vi "XIPIN_100G_Ethernet_1_8.vi"   [LabVIEW 2017]
doc: "The integrated 100G Ethernet IP core provides a 100G Ethernet MAC and PCS/PMA in CAUI-4, CAUI-10, or switchable CAUI-4/CAUI-10 modes, designed to the IEEE 802.3 specification. The IP supports an optional AXI4-Lite interface to access the control and status registers, high accuracy IEEE 1588v2 1-step and 2-step hardware time stamping, and a fee based IEEE 802.3bj RS-FEC core in CAUI-4 mode. For access to the integrated 100G Ethernet MAC IP, please generate a no charge license key from the 100G Ethernet product page. For access to the 100G RS-FEC core, please visit the RS-FEC product page (http://www.xilinx.com/products/intellectual-property/ef-di-100g-rs-fec.html).\n------------------------------------\n<b>Need License</b> : Yes\n<b>Interface</b> : AXI4"
uses:
  <vilib>/rvi/XilinxIP/XIPIN_XNode/niFpgaXIPIN.xnode
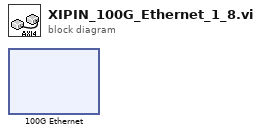
[diagram p0: block diagram]
diagram:
  n1 = xnode ("100G Ethernet")() -> ()
